vi "SkipIfLabVIEWVersionIsIncompatible.vi"(8 "error in (no error)":errorcluster, 10 "Minimum Version Year (2015)":string="2015", 11 "VeriStandTestCase in":refnum<class "VeriStandTestCase.lvclass">) -> (0 "error out":errorcluster, 3 "VeriStandTestCase out":refnum<class "VeriStandTestCase.lvclass">)   [LabVIEW 2015, in "VeriStandTestCase.lvclass"]
uses:
  VeriStandTestCase.lvclass
  VeriStandTestCase.lvclass/VeriStandTestCase.ctl
  <vilib>/addons/_JKI Toolkits/VI Tester/TestCase.llb/TestCase.lvclass
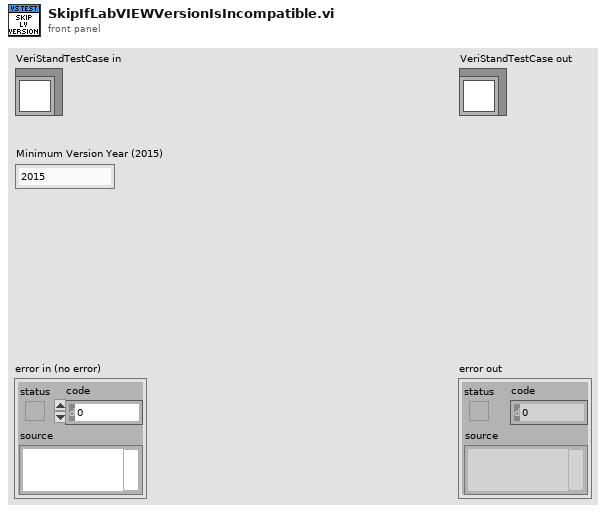
[diagram p1: front panel]
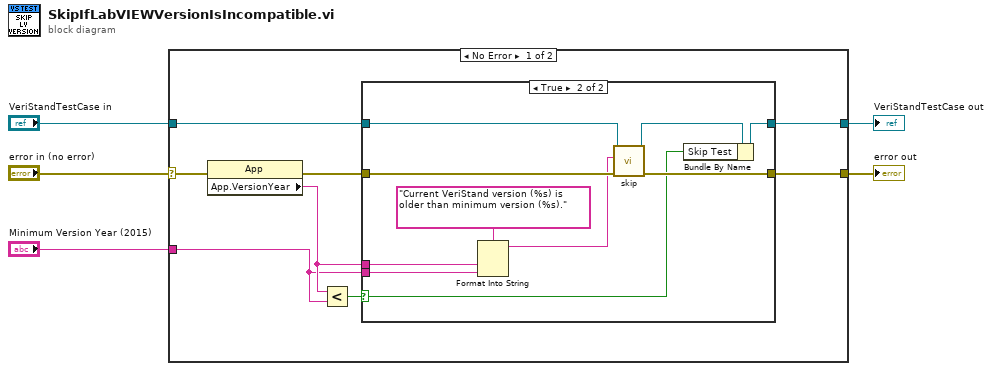
[diagram p0: block diagram]
diagram:
  n1 = case shown="No Error" "error in (no error)" {
    selector: "error in (no error)" -> [w9 w27]
    tunnel: [w7 w27] -> w4
    tunnel: [w10 w26] -> w2
    tunnel: "VeriStandTestCase in" -> [w11 w26]
    tunnel: "Minimum Version Year (2015)" -> [w6 _]
    frame No Error {
      n2 = property class="App"(error in=w9) -> (error out=w8:errorcluster, "App.VersionYear"=w12:string)  [unwired: 1 in, 1 out]
      n3 = Less?(x=w12, y=w6) -> (x < y?=w13:bool)
      n4 = case shown="True" w13 {
        selector: w13 -> [_ w16]
        tunnel: w8 -> [w14 w25]
        tunnel: [w14 w24] -> w7
        tunnel: w11 -> [w15 w23]
        tunnel: [w15 w17] -> w10
        tunnel: w12 -> [_ w20]
        tunnel: w6 -> [_ w19]
        frame False {
        }
        frame True {
          n5 = Format Into String(format string="Current VeriStand version (%s) is older than minimum version (%s).", w20, w19) -> (resulting string=w21:string)  [unwired: 2 in, 1 out]
          n6 = call <vilib>:"skip.vi"("error in (no error)"=w25, "skipMessage"=w21, "TestCase in"=w23) -> ("error out"=w24:errorcluster, "TestCase out"=w18:refnum<class "VeriStandTestCase.lvclass">)  [unwired: 7 in]
          n7 = Bundle By Name(cluster=w18, "Skip Test"=w16) -> (w17:refnum<class "VeriStandTestCase.lvclass">)
        }
      }
    }
    frame Error {
    }
  }
  "error out" <- w4
  "VeriStandTestCase out" <- w2
